vi "Matches.vi"(8 "error in (no error)":errorcluster, 10 "Actual":variant, 11 "Error in":refnum<class "Error.lvclass">) -> (0 "error out":errorcluster, 2 "Result":bool, 3 "Error out":refnum<class "Error.lvclass">)   [LabVIEW 2017, in "Transparent Assertions.lvlib" / "Error.lvclass"]
doc: "Evaluates the constraint for <B>Actual</B>. Returns true if the constraint is met."
uses:
  Error.lvclass
  Error.lvclass/Error.ctl
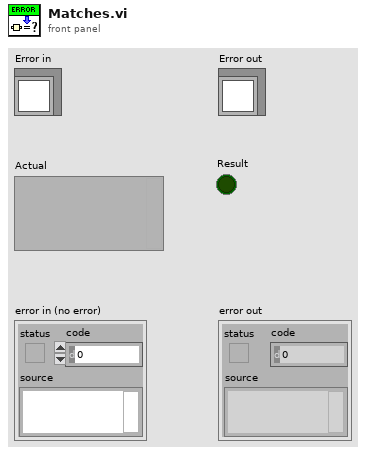
[diagram p1: front panel]
types:
  T1 = typedef "Transparent Assertions.lvlib/Error.lvclass/ErrorType.ctl" = enum16{"error", "warning", "no error"}
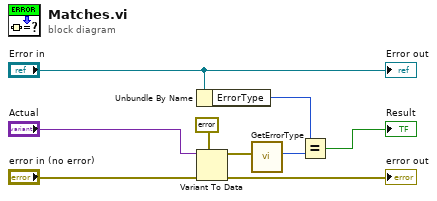
[diagram p0: block diagram]
diagram:
  n1 = Unbundle By Name("Error in") -> ("ErrorType"=w1:T1)
  n2 = Variant To Data(error in="error in (no error)", type=errorcluster {"status"=FALSE, "code"=0, "source"=""} ("error constant"), Variant="Actual") -> (data=w5:errorcluster, error out=→"error out":errorcluster)
  n3 = call "GetErrorType.vi"("error in (no error)"=w5) -> ("ErrorType"=w3:T1)  [unwired: 10 in]
  n4 = Equal?(x=w1, y=w3) -> (x = y?=→"Result":bool)
  "Error out" <- "Error in"
